vi "Global_bits.vi"() -> ()   [LabVIEW 2015]
panel:
  out "Bits":i16[](array[numeric])
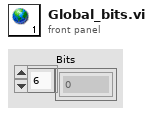
[diagram p1: front panel]
diagram:
